vi "provaJson.vi"() -> ()   [LabVIEW 2010, in "chaosui-crest.lvlib"]
uses:
  chaosui-crest.lvlib
panel:
  out "match substring":string
  in  "channame":string
  out "timestamp":u64
  out "value":cluster{string}
  in  "String":string
  out "error out":errorcluster
  in  "JSON string":string
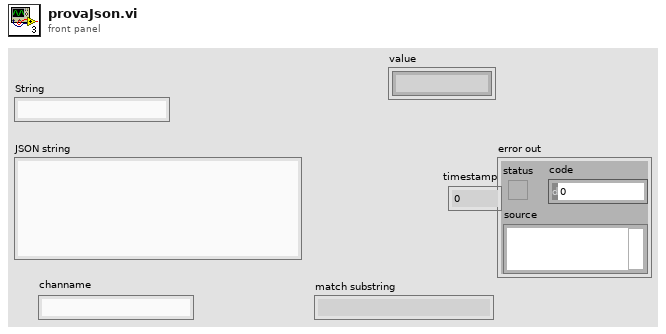
[diagram p1: front panel]
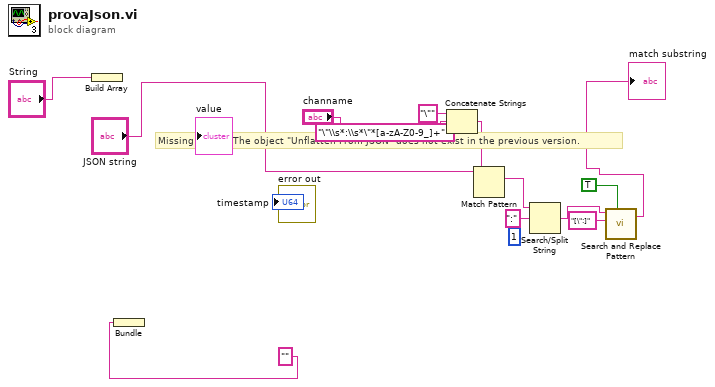
[diagram p0: block diagram]
diagram:
  (unwired) 1 ("offset (0)")
  # "Missing object. The object \"Unflatten From JSON\" does not exist in the previous version."
  n1 = Build Array("String") -> (w14:string[])
  n2 = Bundle("") -> (w15:cluster{string})  [unwired: 1 in]
  n3 = Concatenate Strings("\"" ("string"), "channame", "\"\\s*:\\s*\"*[a-zA-Z0-9_]+" ("string")) -> (w9:string)
  n4 = Match Pattern(string="JSON string", regular expression=w9) -> (match substring=w5:string)  [unwired: 1 in, 3 out]
  n5 = Search/Split String(string=w5, search string/char (-)=":") -> (match + rest of string=w1:string)  [unwired: 1 in, 2 out]
  n6 = call <vilib>:"Search and Replace Pattern.vi"("string"=w1, "regular expression (\"\")"="[\":]" ("regular expression (\"\")"), "replace all? (F)"=TRUE) -> ("result string"=→"match substring":string)  [unwired: 2 in, 1 out]
